vi "VI Tree.vi"   [LabVIEW 2014, in "Associated Research SC6540.lvlib"]
doc: "This is the instrument driver for the ARI38xx LV Instrument Driver, this driver supports the Associated Research 3805, 3855, 3865, 3870, 3880 Electrical Safety Compliance Analyzers. The VI Tree displays all the user-callable VIs of the instrument driver in an organized table.\n\nCreated By: Associated Research, Inc\n13860 West Laurel Drive\nLake Forest, IL 60045\n(847) 367-4077\n(800) 858-8378\n(847) 367-4080 (fax)\nwww.asresearch.com"
uses:
  <instrlib>/Associated Research SC6540/Associated Research SC6540.lvlib
panel:
  # "(c) 2023 IKONIX Group.  ALL RIGHTS RESERVED."
  # "Please see diagram for ARI 38XX Driver VI Tree"
  # "Associated Research\nAn Ikonix Brand\n\n28105 N. Keith Drive\nLake Forest, IL 60045 USA\n\nToll Free:  1-800-858-8378\nPhone:      1-847-367-4077\nFax:          1-847-367-4080\nEmail:        info@ikonix.com"
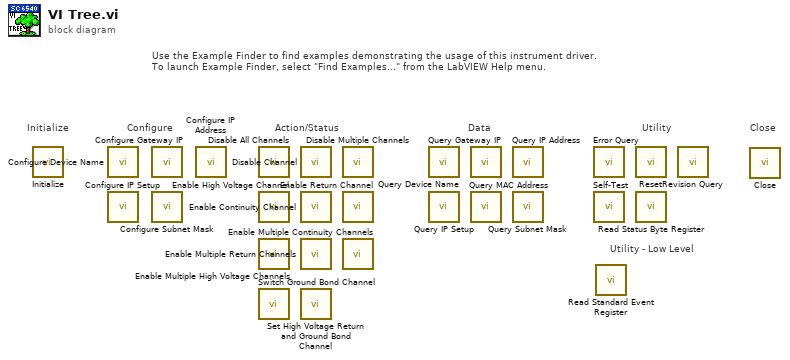
[diagram p0: block diagram]
diagram:
  # "Utility - Low Level"
  # "Data"
  # "Configure"
  # "Close"
  # "Utility"
  # "Use the Example Finder to find examples demonstrating the usage of this instrument driver.\nTo launch Example Finder, select \"Find Examples...\" from the LabVIEW Help menu."
  # "Initialize"
  # "Action/Status"
  n1 = call <instrlib>:"Initialize.vi"() -> ()  [unwired: 10 in, 2 out]
  n2 = call <instrlib>:"Configure Device Name.vi"() -> ()  [unwired: 10 in, 2 out]
  n3 = call <instrlib>:"Configure IP Setup.vi"() -> ()  [unwired: 10 in, 2 out]
  n4 = call <instrlib>:"Configure Gateway IP.vi"() -> ()  [unwired: 10 in, 2 out]
  n5 = call <instrlib>:"Configure Subnet Mask.vi"() -> ()  [unwired: 10 in, 2 out]
  n6 = call <instrlib>:"Configure IP Address.vi"() -> ()  [unwired: 10 in, 2 out]
  n7 = call <instrlib>:"Disable All Channels.vi"() -> ()  [unwired: 10 in, 2 out]
  n8 = call <instrlib>:"Enable High Voltage Channel.vi"() -> ()  [unwired: 10 in, 2 out]
  n9 = call <instrlib>:"Enable Multiple High Voltage Channels.vi"() -> ()  [unwired: 10 in, 2 out]
  n10 = call <instrlib>:"Switch Ground Bond Channel.vi"() -> ()  [unwired: 10 in, 2 out]
  n11 = call <instrlib>:"Disable Channel.vi"() -> ()  [unwired: 10 in, 2 out]
  n12 = call <instrlib>:"Enable Continuity Channel.vi"() -> ()  [unwired: 10 in, 2 out]
  n13 = call <instrlib>:"Enable Multiple Return Channels.vi"() -> ()  [unwired: 10 in, 2 out]
  n14 = call <instrlib>:"Set High Voltage Return and Ground Bond Channel.vi"() -> ()  [unwired: 10 in, 2 out]
  n15 = call <instrlib>:"Disable Multiple Channels.vi"() -> ()  [unwired: 10 in, 2 out]
  n16 = call <instrlib>:"Enable Return Channel.vi"() -> ()  [unwired: 10 in, 2 out]
  n17 = call <instrlib>:"Enable Multiple Continuity Channels.vi"() -> ()  [unwired: 10 in, 2 out]
  n18 = call <instrlib>:"Query Device Name.vi"() -> ()  [unwired: 9 in, 3 out]
  n19 = call <instrlib>:"Query IP Setup.vi"() -> ()  [unwired: 9 in, 3 out]
  n20 = call <instrlib>:"Query Gateway IP.vi"() -> ()  [unwired: 9 in, 3 out]
  n21 = call <instrlib>:"Query MAC Address.vi"() -> ()  [unwired: 9 in, 3 out]
  n22 = call <instrlib>:"Query IP Address.vi"() -> ()  [unwired: 9 in, 3 out]
  n23 = call <instrlib>:"Query Subnet Mask.vi"() -> ()  [unwired: 9 in, 3 out]
  n24 = call <instrlib>:"Error Query.vi"() -> ()  [unwired: 8 in, 4 out]
  n25 = call <instrlib>:"Self-Test.vi"() -> ()  [unwired: 8 in, 4 out]
  n26 = call <instrlib>:"Read Standard Event Register.vi"() -> ()  [unwired: 9 in, 3 out]
  n27 = call <instrlib>:"Reset.vi"() -> ()  [unwired: 10 in, 2 out]
  n28 = call <instrlib>:"Read Status Byte Register.vi"() -> ()  [unwired: 6 in, 6 out]
  n29 = call <instrlib>:"Revision Query.vi"() -> ()  [unwired: 8 in, 4 out]
  n30 = call <instrlib>:"Close.vi"() -> ()  [unwired: 11 in, 1 out]
